vi "init.vi"(8 "error in (no error)":errorcluster, 11 "MotorTemperatureSensor in":refnum<class "MotorTemperatureSensor.lvclass">) -> (0 "error out":errorcluster, 3 "MotorTemperatureSensor out":refnum<class "MotorTemperatureSensor.lvclass">)   [LabVIEW 2013, in "MotorTemperatureSensor.lvclass"]
uses:
  MotorTemperatureSensor.lvclass
  Configuration/Motor Temperature Sensor.ctl
  <userlib>/Common/SerialProtocols/Configuration/SerialConfig.ctl
  <userlib>/Common/SerialProtocols/Configuration/SerialProtocol.ctl
  <userlib>/Common/SerialProtocols/Configuration/ProtocolParameters.ctl
  <userlib>/Common/SerialProtocols/Configuration/SerialMessageParameters.ctl
  Configuration/MotorOverheatTemperature.ctl
  TemperatureSensor/TemperatureSensor.lvclass/TemperatureSensor.ctl
  MotorTemperatureSensor.lvclass/MotorTemperatureSensor.ctl
  ConfigurationThisComponent/ConfigurationThisComponent.lvclass
  TemperatureSensor/TemperatureSensor.lvclass
  <userlib>/Common/SerialProtocols/SerialProtocols.lvlib
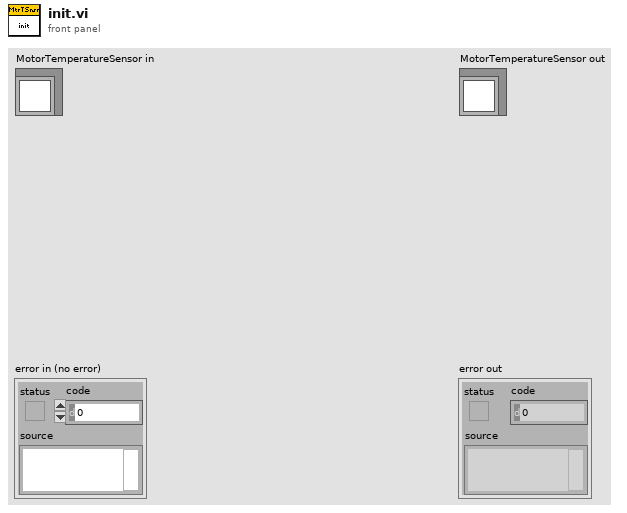
[diagram p1: front panel]
types:
  T1 = typedef "Motor Temperature Sensor.ctl" = cluster{"Serial":T2, "Motor Overheat Temperature":T6}
  T2 = typedef "SerialProtocols.lvlib/SerialConfig.ctl" = cluster{"Serial Protocol":T3, "Protocol Parameters":T4, "Serial Message Parameters":T5}
  T3 = typedef "SerialProtocols.lvlib/SerialProtocol.ctl" = enum16{"RS232", "RS485", "SerialSimulator"}
  T4 = typedef "SerialProtocols.lvlib/ProtocolParameters.ctl" = cluster{"VISA resource name":refnum<visa-resource-name>, "Baud Rate":u32, "Data Bits":u16, "Parity":enum16{"None", "Odd", "Even", "Mark", "Space"}, "Flow Control":u16, "Stop Bits":u16, "Timeout (ms)":u32}
  T5 = typedef "SerialProtocols.lvlib/SerialMessageParameters.ctl" = cluster{"Byte Count":u32, "Enable Termination Character":bool, "Termination Char":u8}
  T6 = typedef "MotorOverheatTemperature.ctl" = dbl[unit]
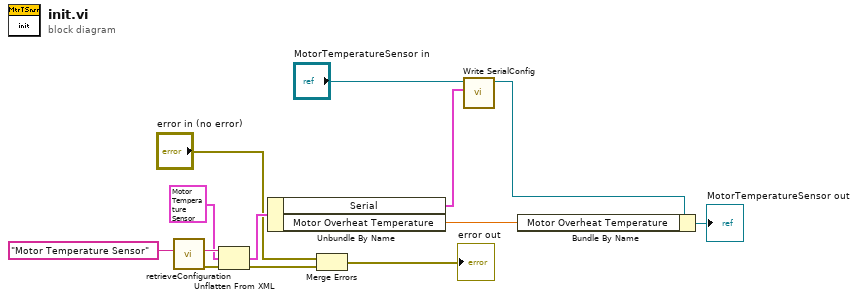
[diagram p0: block diagram]
diagram:
  n1 = call "retrieveConfiguration.vi"("configName"="Motor Temperature Sensor") -> ("error out"=w10:errorcluster, "xmlConfig"=w11:string)  [unwired: 8 in, 1 out]
  n2 = Unflatten From XML(xml string=w11, type=T1 {"Serial"={"Serial Protocol"=enum."RS232", "Protocol Parameters"={"VISA resource name"="", "Baud Rate"=0, "Data Bits"=0, "Parity"=enum."None", "Flow Control"=0, "Stop Bits"=0, "Timeout (ms)"=0}, "Serial Message Parameters"={"Byte Count"=0, "Enable Termination Character"=FALSE, "Termination Char"=0}}, "Motor Overheat Temperature"=0.0} ("Motor Temperature Sensor"), error in (no error)=w10) -> (value=w9:T1, error out=w13:errorcluster)
  n3 = Unbundle By Name(w9) -> ("Serial"=w8:T2, "Motor Overheat Temperature"=w2:T6)
  n4 = Merge Errors("error in (no error)", w13) -> (→"error out":errorcluster)
  n5 = call "Write SerialConfig.vi"("SerialConfig"=w8, "TemperatureSensor in"="MotorTemperatureSensor in") -> ("TemperatureSensor out"=w3:refnum<class "MotorTemperatureSensor.lvclass">)  [unwired: 9 in]
  n6 = Bundle By Name(cluster=w3, "Motor Overheat Temperature"=w2) -> (→"MotorTemperatureSensor out":refnum<class "MotorTemperatureSensor.lvclass">)
